vi "WheeTrometerChrom.vi"() -> ()   [LabVIEW 2020]
uses:
  <vilib>/Native 3D Graph/xcontrol/3DPC_SurfacePlot.xctl
  <vilib>/Analysis/baseanly.llb/Mean (DBL).vi
  <vilib>/Instr/_visa.llb/VISA Configure Serial Port (Instr).vi
  WheeChromGlobals.vi
  <vilib>/Analysis/NI_AALBase.lvlib
  <vilib>/Platform/NI_3dgraph.lvlib
panel:
  out "Connection":bool
  in  "Tab Control":enum32{"Chrom Data", "Spectrometer Settings"}(tab)
  in  "3D Surface":refnum<k7>(container)
  out "XY Graph 2":cluster{"WavelengthCal":dbl[], "Array":i32[]}(graph)
  out "Chromatogram at wavelength of interest":i32[](graph)
  in  "Start":bool
  in  "Length of Chromatogram (sec)":dbl
  in  "wavelength of interest":dbl
  out "Total Chromatogram":refnum<class "Base Datatype.lvclass">[](xcontrol)
  in  "file path (use dialog)":path
  out "XY Graph":cluster{"WavelengthCal":dbl[], "Array":i32[]}(graph)
  in  "Single Spec":bool
  in  "spectra to average (per spec)":dbl
  in  "pixels to average (per spec)":dbl
  in  "Intergratin time (ms) (per spec)":dbl
  in  "Initiate":bool
  out "VISA resource name out":refnum<visa-resource-name>
  out "A":dbl
  out "B":dbl
  out "C":dbl
  out "+":dbl
  out "=":dbl
  in  "Auto Find":bool
  in  "reference":refnum<visa-resource-name>
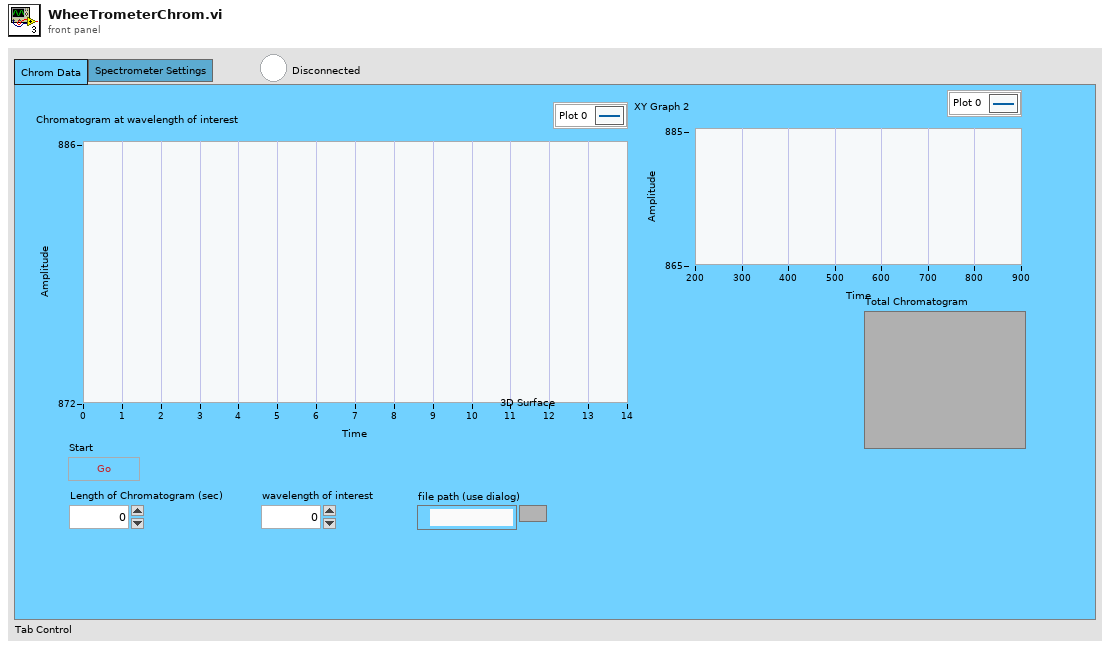
[diagram p1: front panel]
types:
  T1 = enum16{"open", "replace", "create", "open or create", "replace or create", "replace or create with confirmation"}
  T2 = enum16{"open", "open or create", "create or replace", "create", "open (read-only)"}
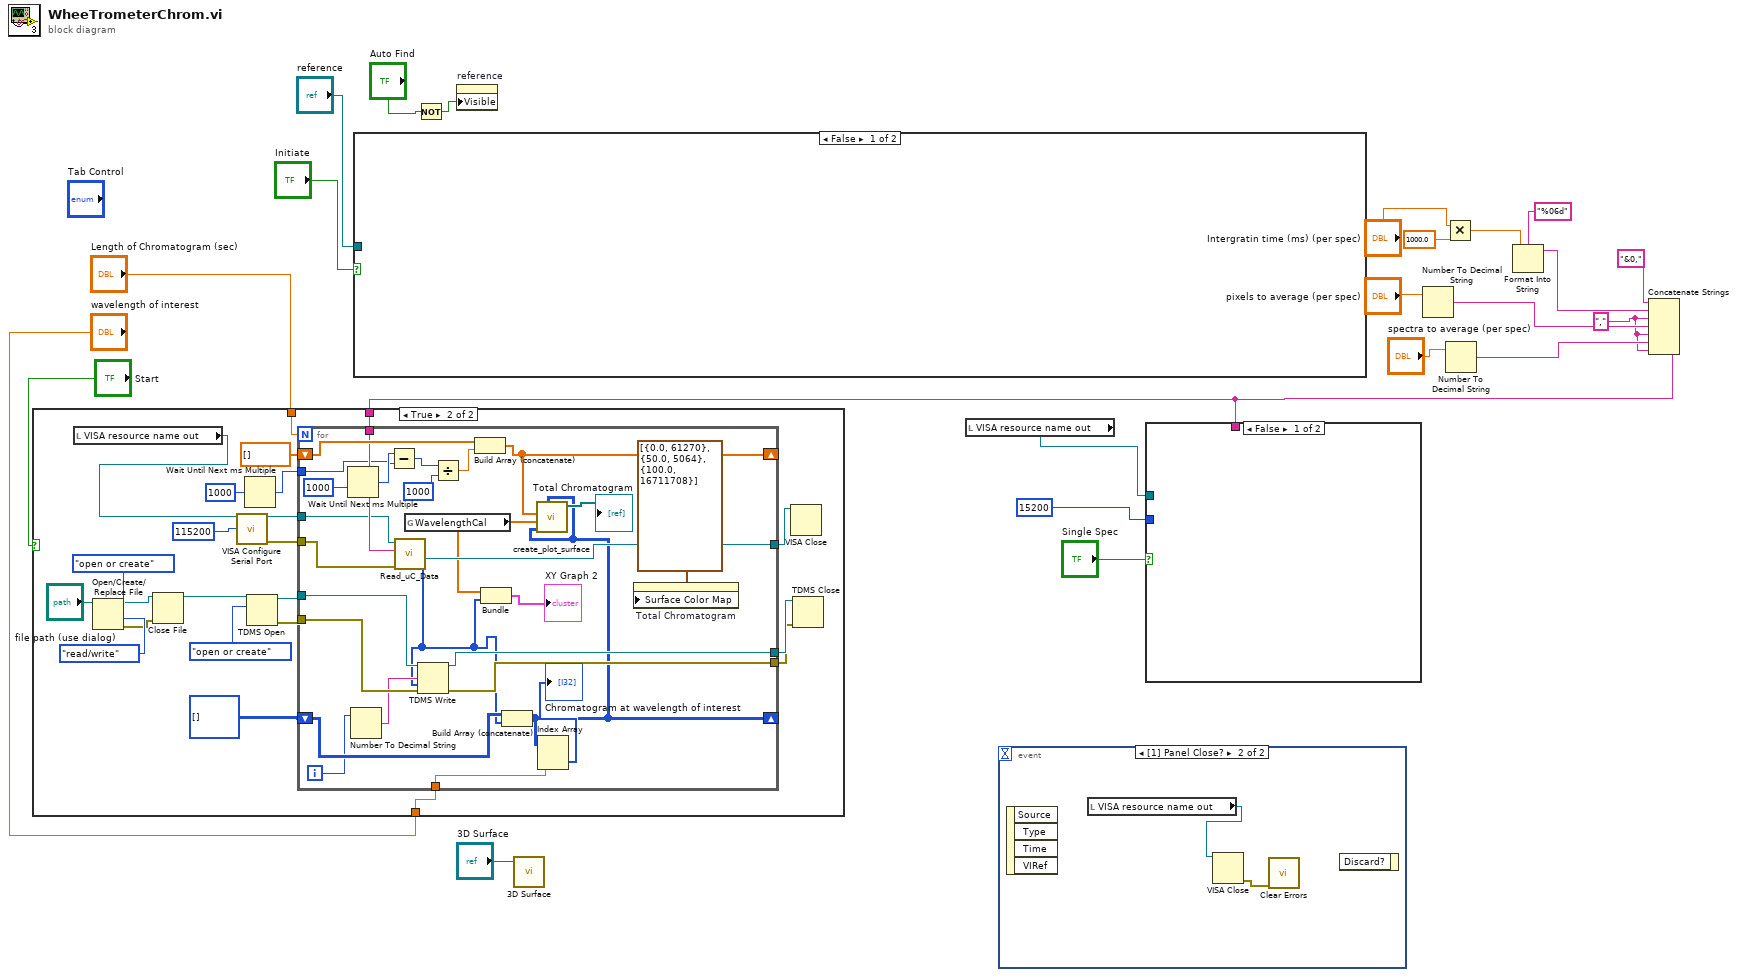
[diagram p0: block diagram]
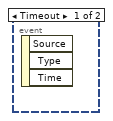
[diagram p2: hidden frame]
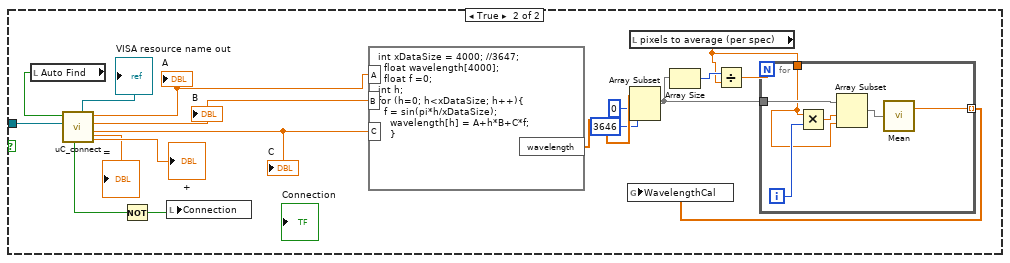
[diagram p3: hidden frame]
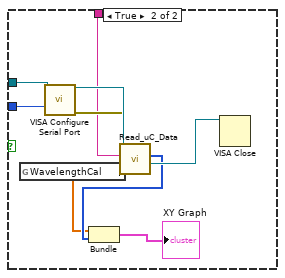
[diagram p5: hidden frame]
diagram:
  w13 = "," ("string")
  n1 = case shown="False" "Initiate" {
    tunnel: "reference" -> [_ w24]
    frame False {
    }
    frame True {
      n2 = local read "Auto Find"() -> (w25:bool)
      n3 = call "uC_connect.vi"("reference"=w24, "find port"=w25) -> ("+"=→"+":dbl, "C"=w37:dbl, "B"=w38:dbl, "A"=w39:dbl, "="=→"=":dbl, "VISA resource name out"=→"VISA resource name out":refnum<visa-resource-name>, "status"=w26:bool)  [unwired: 2 in, 1 out]
      "A" <- w39
      "B" <- w38
      "C" <- w37
      n4 = Not(x=w26) -> (.not. x?=w27:bool)
      n5 = local write "Connection"(w27) -> ()
      n6 = formula code="int xDataSize = 4000; //3647;                \n  float wavelength[4000];\n  float f =0;\nint h;\nfor (h=0; h<xDataSize; h++){\n  f = sin(pi*h/xDataSize);\n    wavelength[h] = A+h*B+C*f;\n    }"("A"=w39, "B"=w38, "C"=w37) -> ("wavelength"=w36:dbl[])
      n7 = local read "pixels to average (per spec)"() -> (w30:dbl)
      n8 = Array Subset(array=w36, index=0, length=3646) -> (w31:dbl[])
      n9 = Array Size(array=w31) -> (size(s)=w33:i32)
      n10 = Divide(x=w33, y=w30) -> (x/y=w32:dbl)
      n11 = for {
        N: w32 -> [_]
        tunnel: w31 -> [w47]
        tunnel: w30 -> [w44]
        tunnel: [w42] -> w29 mode=indexing
        i -> [w45]
        n12 = Multiply(x=w44, y=w45) -> (x*y=w46:dbl)
        n13 = Array Subset(array=w47, index=w46, length=w44) -> (w43:dbl[])
        n14 = call-poly <vilib>:"Mean.vi"("X"=w43) -> ("mean"=w42:dbl)  [unwired: 1 out]
      }
      n15 = global write "WheeChromGlobals.vi" "WavelengthCal"(w29) -> ()
    }
  }
  n16 = Not(x="Auto Find") -> (.not. x?=w4:bool)
  n17 = property on="reference" class="VISAName"("Visible"=w4) -> ()  [unwired: 2 in, 2 out]
  n18 = call <vilib>:"3D Surface.vi"("3D graph"="3D Surface") -> ()  [unwired: 9 in, 2 out]
  n19 = local read "VISA resource name out"() -> (w6:refnum<visa-resource-name>)
  n20 = event shown="[1] Panel Close?" {
    selector: _ -> [_ _]
    dyn-events: _ -> [_ _]
    timeout: _ -> [_ _]
    event Timeout {
      n21 = event-data() -> ()  [unwired: 1 in, 3 out]
    }
    event Panel Close? {
      n22 = event-data() -> ()  [unwired: 1 in, 4 out]
      n23 = local read "VISA resource name out"() -> (w49:refnum<visa-resource-name>)
      n24 = VISA Close(VISA resource name=w49) -> (error out=w48:errorcluster)  [unwired: 1 in]
      n25 = call <vilib>:"Clear Errors.vi"("error in (no error)"=w48) -> ()  [unwired: 5 in, 2 out]
      n26 = event-data() -> ()  [unwired: 2 in, 1 out]
    }
  }
  n27 = Number To Decimal String(number="pixels to average (per spec)") -> (decimal integer string=w15:string)  [unwired: 1 in]
  n28 = Multiply(x="Intergratin time (ms) (per spec)", y=1000.0) -> (x*y=w22:dbl)
  n29 = Number To Decimal String(number="spectra to average (per spec)") -> (decimal integer string=w14:string)  [unwired: 1 in]
  n30 = Format Into String(format string="%06d", w22) -> (resulting string=w16:string)  [unwired: 2 in, 1 out]
  n31 = Concatenate Strings("&0," ("string"), w16, w13, w15, w13, w14, w13) -> (w11:string)
  n32 = case shown="True" "Start" {
    tunnel: w11 -> [_ w70]
    tunnel: "Length of Chromatogram (sec)" -> [_ w69]
    tunnel: "wavelength of interest" -> [_ w67]
    frame False {
    }
    frame True {
      n33 = local read "VISA resource name out"() -> (w53:refnum<visa-resource-name>)
      n34 = Open/Create/Replace File(file path (use dialog)="file path (use dialog)", operation (0:open)=T1."open or create", access (0:read/write)=enum16{"read/write", "read-only", "write-only"}."read/write") -> (refnum out=w56:refnum<file>, error out=w57:errorcluster)  [unwired: 3 in, 1 out]
      n35 = Close File(refnum=w56, error in=w57) -> (path=w55:path)  [unwired: 1 out]
      n36 = call-poly "VISA Configure Serial Port"("VISA resource name"=w53, "baud rate (9600)"=u32 115200) -> ("VISA resource name out"=w72:refnum<visa-resource-name>, "error out"=w71:errorcluster)  [unwired: 12 in]
      n37 = Wait Until Next ms Multiple(millisecond multiple=u32 1000) -> (millisecond timer value=w50:u32)
      n38 = TDMS Open(10:T2."open or create" ("operation (0:open)"), 11:w55) -> (0:w61:errorcluster, 3:w60:refnum<k34>)  [unwired: 5 in]
      n39 = for {
        N: w69 -> [_]
        tunnel: w72 -> [w90]
        tunnel: w71 -> [w89]
        tunnel: w70 -> [w91]
        shift-right: [w76] -> _
        shift-left: i32[][] [] -> [w98]
        tunnel: w67 -> [w96]
        shift-right: [w92] -> _
        shift-left: dbl[] [] -> [w93]
        tunnel: [w87] -> w65
        tunnel: [w85] -> w64
        tunnel: [w84] -> w63
        tunnel: w61 -> [w83]
        tunnel: w60 -> [w82]
        tunnel: w50 -> [w73]
        i -> [w81]
        n40 = Wait Until Next ms Multiple(millisecond multiple=u32 1000) -> (millisecond timer value=w74:u32)
        n41 = Number To Decimal String(number=w81) -> (decimal integer string=w80:string)  [unwired: 1 in]
        n42 = Subtract(x=w74, y=w73) -> (x-y=w75:u32)
        n43 = call "Read_uC_Data.vi"("error in (no error)"=w89, "String"=w91, "VISA Refnum in"=w90) -> ("VISA Refnum in 2"=w87:refnum<visa-resource-name>, "Array"=w78:i32[])  [unwired: 6 in, 1 out]
        n44 = global read "WheeChromGlobals.vi" "WavelengthCal"() -> (w77:dbl[])
        n45 = TDMS Write(0:w82, 7:w80, 9:w78, 11:w83) -> (4:w85:refnum<k34>, 15:w84:errorcluster)  [unwired: 2 in, 2 out]
        n46 = Divide(x=w75, y=u32 1000) -> (x/y=w94:dbl)
        n47 = Build Array (concatenate)(w93, w94) -> (w92:dbl[])
        n48 = Bundle("WavelengthCal"=w77, "Array"=w78) -> (→"XY Graph 2":cluster{"WavelengthCal":dbl[], "Array":i32[]})  [unwired: 1 in]
        n49 = Build Array (concatenate)(w98, w78) -> (w76:i32[][])
        n50 = call <vilib>:"create_plot_surface.vi"("color matrix"=w76, "z matrix"=w76, "y vector"=w77, "x vector"=w92) -> ("plots out"=→"Total Chromatogram":refnum<class "Base Datatype.lvclass">[])  [unwired: 2 in, 5 out]
        n51 = Index Array(array=w76, index (col)=w96) -> (element=→"Chromatogram at wavelength of interest":i32[])  [unwired: 1 in]
        n52 = property on="Total Chromatogram" class="LabVIEW 3D Graph (strict)"("Surface Color Map"=cluster{dbl, u32}[] [{0.0, 61270}, {50.0, 5064}, {100.0, 16711708}] ("Plots:Surface Color Map")) -> ()  [unwired: 2 in, 2 out]
      }
      n53 = VISA Close(VISA resource name=w65) -> ()  [unwired: 1 in, 1 out]
      n54 = TDMS Close(8:w63, 11:w64) -> ()  [unwired: 2 out]
    }
  }
  n55 = case shown="False" "Single Spec" {
    tunnel: w11 -> [_ w106]
    tunnel: u32 15200 ("baud rate (9600)") -> [_ w105]
    tunnel: w6 -> [_ w104]
    frame False {
    }
    frame True {
      n56 = global read "WheeChromGlobals.vi" "WavelengthCal"() -> (w100:dbl[])
      n57 = call-poly "VISA Configure Serial Port"("VISA resource name"=w104, "baud rate (9600)"=w105) -> ("VISA resource name out"=w108:refnum<visa-resource-name>, "error out"=w107:errorcluster)  [unwired: 12 in]
      n58 = call "Read_uC_Data.vi"("error in (no error)"=w107, "String"=w106, "VISA Refnum in"=w108) -> ("VISA Refnum in 2"=w103:refnum<visa-resource-name>, "Array"=w102:i32[])  [unwired: 6 in, 1 out]
      n59 = Bundle("WavelengthCal"=w100, "Array"=w102) -> (→"XY Graph":cluster{"WavelengthCal":dbl[], "Array":i32[]})  [unwired: 1 in]
      n60 = VISA Close(VISA resource name=w103) -> ()  [unwired: 1 in, 1 out]
    }
  }
